vi "OPEN.vi"(11 "Pump_1AI_1DO_2DI in":refnum<class "NeedleValve.lvclass">) -> (3 "Pump_1AI_1DO_2DI out":refnum<class "NeedleValve.lvclass">)   [LabVIEW 2019]
uses:
  TypeDef/Needle Valve State.ctl
  NeedleValve.lvclass
  D:/GIT H4000/H4000/src/Device_class/Device.lvclass
  D:/GIT H4000/H4000/src/Proccess_class/Proccess.lvclass
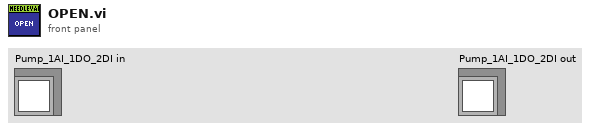
[diagram p1: front panel]
types:
  T1 = typedef "Needle Valve State.ctl" = enum16{"IDLE", "OPEN", "CLOSE", "OPENING", "CLOSING", "STOP"}
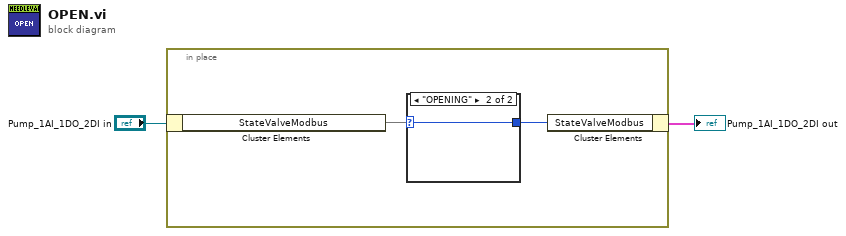
[diagram p0: block diagram]
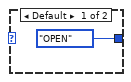
[diagram p2: hidden frame]
diagram:
  n1 = in-place {
    n2 = in-place-cluster #1("Pump_1AI_1DO_2DI in") -> ("StateValveModbus"=w4)
    n3 = case shown="\"OPENING\"" w4 {
      selector: w4 -> [_ w6]
      tunnel: [Needle_Valve_State."OPEN" ("StateValveModbus") w6] -> w3
      frame Default {
      }
      frame "OPENING" {
      }
    }
    n4 = in-place-cluster #1("StateValveModbus"=w3) -> (→"Pump_1AI_1DO_2DI out":cluster{})
  }
